vi "WPI_CameraIssue HTTP Request with Authentication.vi"(7 "port":u16=80, 8 "error in (no error)":errorcluster, 9 "Authenticate":bool=TRUE, 10 "Request":string, 11 "address":string) -> (0 "error out":errorcluster, 2 "Authenticated request":string, 3 "connection ID (dup)":refnum<k5>)   [LabVIEW 2017]
doc: "This VI issues the given http request with the required added information and authentication. It cycles through an array of predetermined username, password combinations that we expect the users to have at any point in time. If none of the username, password combinations work, this VI returns an \"Unknown user or password\" error.\n\nThis software is licensed. Open the labview\\readme\\WPI Robotics Library Open Source License.txt file for more information."
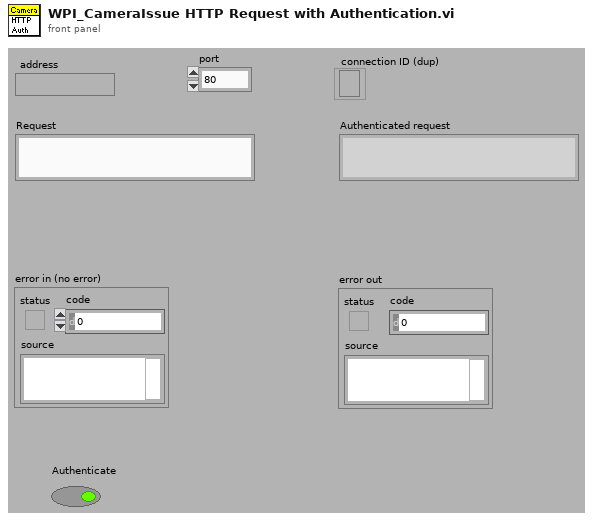
[diagram p1: front panel]
types:
  T1 = enum16{"Standard", "Buffered", "CRLF", "Immediate"}
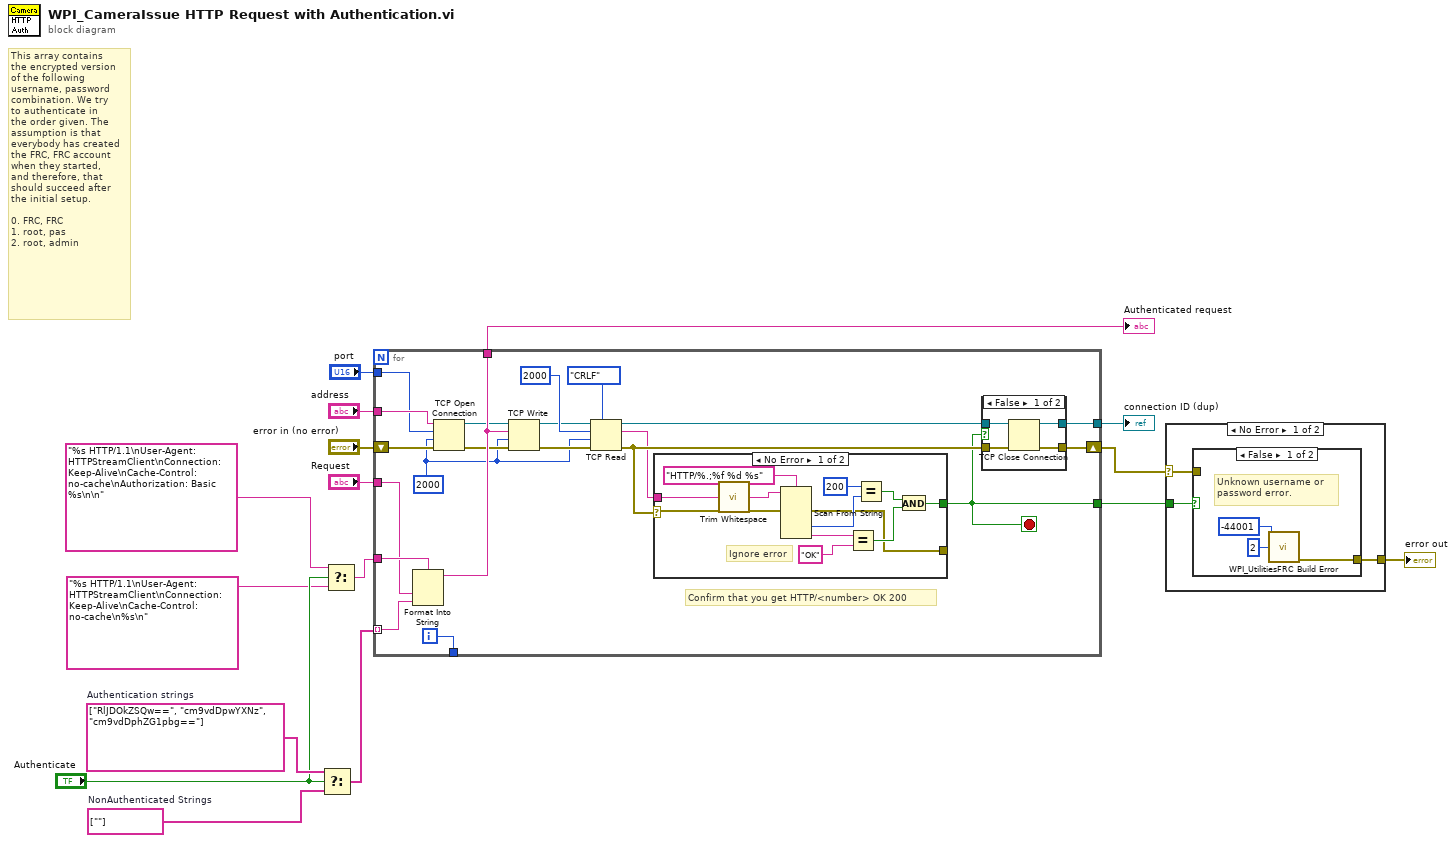
[diagram p0: block diagram]
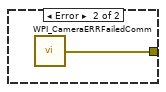
[diagram p3: hidden frame]
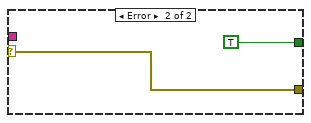
[diagram p5: hidden frame]
diagram:
  w5 = string[] [""]  # NonAuthenticated Strings
  w7 = string[] ["RlJDOkZSQw==", "cm9vdDpwYXNz", "cm9vdDphZG1pbg=="]  # Authentication strings
  # "This array contains\nthe encrypted version\nof the following \nusername, password\ncombination. We try \nto authenticate in\nthe order given. The \nassumption is that \neverybody has created\nthe FRC, FRC account\nwhen they started,\nand therefore, that\nshould succeed after\nthe initial setup.\n\n0. FRC, FRC\n1. root, pas\n2. root, admin"
  n1 = Select(t=w7, s="Authenticate", f=w5) -> (s? t:f=w6:string[])
  n2 = Select(t="%s HTTP/1.1\nUser-Agent: HTTPStreamClient\nConnection: Keep-Alive\nCache-Control: no-cache\nAuthorization: Basic %s\n\n", s="Authenticate", f="%s HTTP/1.1\nUser-Agent: HTTPStreamClient\nConnection: Keep-Alive\nCache-Control: no-cache\n%s\n") -> (s? t:f=w3:string)
  n3 = for {
    shift-right: [w22] -> w14
    shift-left: "error in (no error)" -> [w28]
    tunnel: w3 -> [w33]
    tunnel: "Request" -> [w32]
    tunnel: w6 -> [w31] mode=indexing
    tunnel: [w24] -> w13
    tunnel: [w30] -> w11
    tunnel: [w23] -> w10
    tunnel: "address" -> [w21]
    tunnel: [w20] -> _
    tunnel: "port" -> [w17]
    i -> [w20]
    stop <- w24 stop-if-true
    w18 = 2000 ("timeout ms (60000)")
    # "Confirm that you get HTTP/<number> OK 200"
    n4 = Format Into String(format string=w33, w32, w31) -> (resulting string=w30:string)  [unwired: 2 in, 1 out]
    n5 = TCP Open Connection(address=w21, remote port or service name=w17, timeout ms (60000)=w18, error in (no error)=w28) -> (connection ID=w29:refnum<k5>, error out=w27:errorcluster)  [unwired: 1 out]
    n6 = TCP Write(connection ID=w29, data in=w30, error in (no error)=w27, 9:w18) -> (connection ID out=w35:refnum<k5>, error out=w34:errorcluster)  [unwired: 1 out]
    n7 = TCP Read(connection ID=w35, bytes to read=2000, error in (no error)=w34, 7:T1."CRLF" ("mode (standard)"), 9:w18) -> (connection ID out=w26:refnum<k5>, data out=w19:string, error out=w25:errorcluster)
    n8 = case shown="No Error" w25 {
      selector: w25 -> [w47 w57]
      tunnel: [w48 TRUE] -> w24
      tunnel: [w46 w57] -> _
      tunnel: w19 -> [w44 _]
      frame No Error {
        # "Ignore error"
        n9 = call <vilib>:"Trim Whitespace.vi"("string"=w44) -> ("trimmed string"=w45:string)  [unwired: 1 in]
        n10 = Scan From String(format string="HTTP/%.;%f %d %s", input string=w45, error in=w47) -> (error out=w46:errorcluster, output 2=w54:i32, output 3=w52:string)  [unwired: 1 in, 6 out]
        n11 = Equal?(x=w52, y="OK" ("format string")) -> (x = y?=w50:bool)
        n12 = Equal?(x=200, y=w54) -> (x = y?=w49:bool)
        n13 = And(x=w49, y=w50) -> (x .and. y?=w48:bool)
      }
      frame Error {
      }
    }
    n14 = case shown="False" w24 {
      tunnel: w26 -> [w41 w43]
      tunnel: w25 -> [w40 w42]
      tunnel: [w39 w43] -> w23
      tunnel: [w38 w42] -> w22
      frame False {
        n15 = TCP Close Connection(connection ID=w41, error in (no error)=w40) -> (connection ID out=w39:refnum<k5>, error out=w38:errorcluster)  [unwired: 1 out]
      }
      frame True {
      }
    }
  }
  "connection ID (dup)" <- w10
  "Authenticated request" <- w11
  n16 = case shown="No Error" w14 {
    selector: w14 -> [w58 _]
    tunnel: w13 -> [w60 _]
    tunnel: [w59 w65] -> w12
    frame No Error {
      n17 = case shown="False" w60 {
        tunnel: [w61 w64] -> w59
        tunnel: w58 -> [_ w64]
        frame False {
          # "Unknown username or\npassword error."
          n18 = call <vilib>:"WPI_UtilitiesFRC Build Error.vi"("error code"=-44001 ("code"), "chain levels to remove (1)"=2) -> ("error out"=w61:errorcluster)  [unwired: 3 in, 10 out]
        }
        frame True {
        }
      }
    }
    frame Error {
      n19 = call <vilib>:"WPI_CameraERRFailedComm.vi"() -> ("error out"=w65:errorcluster)
    }
  }
  "error out" <- w12
